vi "Find current file num.vi"() -> (0 "Current File Num":u16)   [LabVIEW 2015]
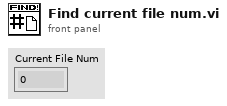
[diagram p1: front panel]
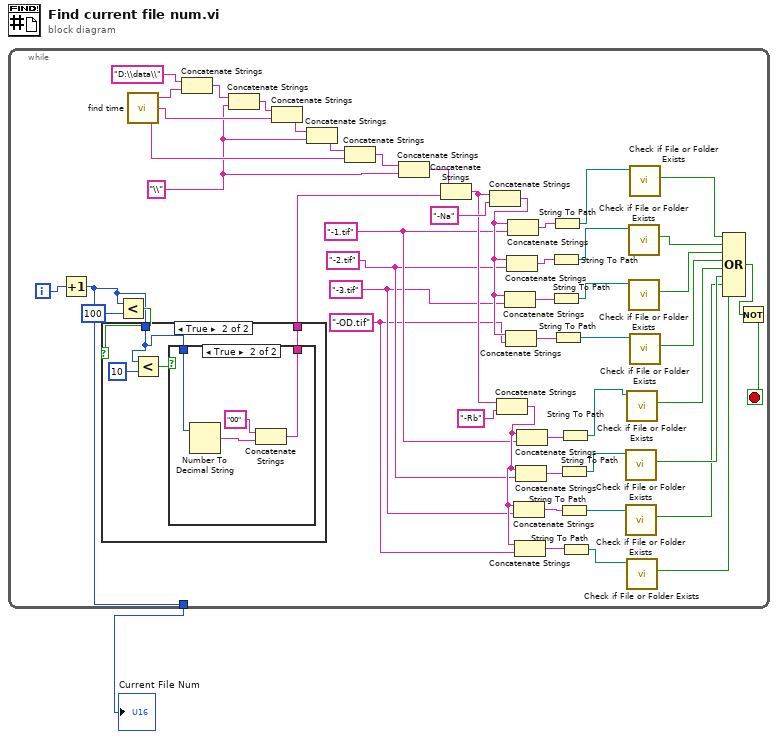
[diagram p0: block diagram]
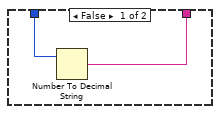
[diagram p2: hidden frame]
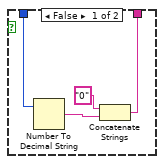
[diagram p3: hidden frame]
diagram:
  n1 = while {
    tunnel: [w25] -> w1
    i -> [w52]
    stop <- w28 stop-if-true
    w18 = "-1.tif" ("字符串")
    w17 = "-2.tif" ("字符串")
    w16 = "-3.tif" ("字符串")
    w15 = "-OD.tif" ("字符串")
    w42 = "\\" ("字符串")
    n2 = Increment(x=w52) -> (x+1=w25:i32)
    n3 = Less?(x=w25, y=100) -> (x < y?=w26:bool)
    n4 = case shown="True" w26 {
      tunnel: w25 -> [w54 w56]
      tunnel: [w53 w55] -> w24
      frame False {
        n5 = Number To Decimal String(number=w54) -> (decimal integer string=w53:string)  [unwired: 1 in]
      }
      frame True {
        n6 = Less?(x=w56, y=10) -> (x < y?=w57:bool)
        n7 = case shown="True" w57 {
          tunnel: w56 -> [w60 w66]
          tunnel: [w59 w63] -> w55
          frame False {
            n8 = Number To Decimal String(number=w60) -> (decimal integer string=w62:string)  [unwired: 1 in]
            n9 = Concatenate Strings("0" ("字符串"), w62) -> (w59:string)
          }
          frame True {
            n10 = Number To Decimal String(number=w66) -> (decimal integer string=w65:string)  [unwired: 1 in]
            n11 = Concatenate Strings("00" ("字符串"), w65) -> (w63:string)
          }
        }
      }
    }
    n12 = call "find time.vi"() -> ("day"=w44:string, "month"=w47:string, "year"=w50:string)  [unwired: 3 in]
    n13 = Concatenate Strings("D:\\data\\", w50) -> (w49:string)
    n14 = Concatenate Strings(w49, w42) -> (w48:string)
    n15 = Concatenate Strings(w48, w47) -> (w46:string)
    n16 = Concatenate Strings(w46, w42) -> (w45:string)
    n17 = Concatenate Strings(w45, w44) -> (w43:string)
    n18 = Concatenate Strings(w43, w42) -> (w41:string)
    n19 = Concatenate Strings(w41, w24) -> (w21:string)
    n20 = Concatenate Strings(w21, "-Na" ("string")) -> (w22:string)
    n21 = Concatenate Strings(w21, "-Rb" ("string")) -> (w19:string)
    n22 = Concatenate Strings(w22, w16) -> (w37:string)
    n23 = Concatenate Strings(w22, w15) -> (w36:string)
    n24 = Concatenate Strings(w22, w17) -> (w38:string)
    n25 = Concatenate Strings(w22, w18) -> (w39:string)
    n26 = Concatenate Strings(w19, w16) -> (w12:string)
    n27 = Concatenate Strings(w19, w15) -> (w11:string)
    n28 = Concatenate Strings(w19, w17) -> (w13:string)
    n29 = Concatenate Strings(w19, w18) -> (w14:string)
    n30 = String To Path(string=w38) -> (path=w35:path)
    n31 = String To Path(string=w37) -> (path=w34:path)
    n32 = String To Path(string=w39) -> (path=w40:path)
    n33 = String To Path(string=w36) -> (path=w33:path)
    n34 = String To Path(string=w13) -> (path=w9:path)
    n35 = String To Path(string=w12) -> (path=w8:path)
    n36 = String To Path(string=w14) -> (path=w10:path)
    n37 = String To Path(string=w11) -> (path=w7:path)
    n38 = call <vilib>:"Check if File or Folder Exists.vi"("path"=w9) -> ("file or folder exists?"=w5:bool)  [unwired: 8 in, 2 out]
    n39 = call <vilib>:"Check if File or Folder Exists.vi"("path"=w8) -> ("file or folder exists?"=w4:bool)  [unwired: 8 in, 2 out]
    n40 = call <vilib>:"Check if File or Folder Exists.vi"("path"=w10) -> ("file or folder exists?"=w6:bool)  [unwired: 8 in, 2 out]
    n41 = call <vilib>:"Check if File or Folder Exists.vi"("path"=w7) -> ("file or folder exists?"=w3:bool)  [unwired: 8 in, 2 out]
    n42 = call <vilib>:"Check if File or Folder Exists.vi"("path"=w35) -> ("file or folder exists?"=w31:bool)  [unwired: 8 in, 2 out]
    n43 = call <vilib>:"Check if File or Folder Exists.vi"("path"=w34) -> ("file or folder exists?"=w30:bool)  [unwired: 8 in, 2 out]
    n44 = call <vilib>:"Check if File or Folder Exists.vi"("path"=w40) -> ("file or folder exists?"=w32:bool)  [unwired: 8 in, 2 out]
    n45 = call <vilib>:"Check if File or Folder Exists.vi"("path"=w33) -> ("file or folder exists?"=w29:bool)  [unwired: 8 in, 2 out]
    n46 = Compound Arithmetic op=OR(w32, w31, w30, w29, w6, w5, w4, w3) -> (w2:bool)
    n47 = Not(x=w2) -> (.not. x?=w28:bool)
  }
  "Current File Num" <- w1
